vi "PDLM_GetDriverServiceName.vi"(11 "error in (no error)":errorcluster) -> (4 "return type":i32, 6 "cName":string, 15 "error out":errorcluster)   [LabVIEW 2017]
doc: "Gets service name of currently installed Taiko driver"
uses:
  PDLM_DllPath_global.vi
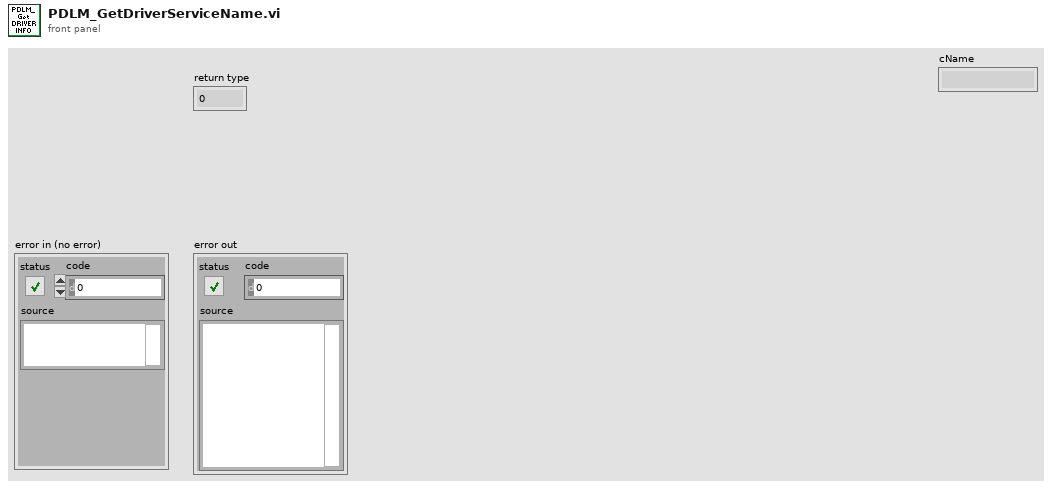
[diagram p1: front panel]
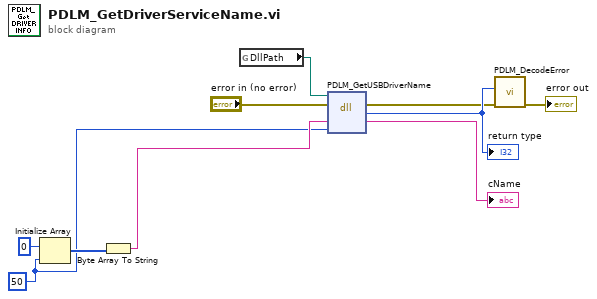
[diagram p0: block diagram]
diagram:
  w1 = 50 ("dimension size")
  n1 = Initialize Array(u8 0 ("element"), w1) -> (w3:u8[])
  n2 = Byte Array To String(unsigned byte array=w3) -> (string=w2:string)
  n3 = global read "PDLM_DllPath_global.vi" "DllPath"() -> (w6:path)
  n4 = dll-call lib="M:/_dev/progs/LabVIEW/_lib/PQ/Taiko/pdlm_lib.dll" fn="PDLM_GetUSBDriverName"(path in=w6, error in="error in (no error)", "cName"=w2, "uiNBuffLen"=w1) -> (error out=w8:errorcluster, "return type"=w9:i32, "cName"=→"cName":string)  [unwired: 2 in, 1 out]
  "return type" <- w9
  n5 = call "PDLM_DecodeError.vi"("error in (no error)"=w8, "code"=w9) -> ("error out"=→"error out":errorcluster)  [unwired: 7 in, 2 out]
